vi "Parameter Analyzer Time-IDX_Download.vi"(2 "Error In (no error)":errorcluster, 3 "Trace (variable) name":string, 4 "VISA session":refnum<visa-resource-name>) -> (0 "Error Out":errorcluster, 1 "Trace":dbl[](array[numeric]) format="%^.3e")   [LabVIEW 2014]
uses:
  <instrlib>/Agilent 415X Series/Agilent 415X Series.lvlib
panel:
  # "LICENSED MATERIALS – PROPERTY OF IBM\nCopyright IBM Corp. 2016,\nALL RIGHTS RESERVED"
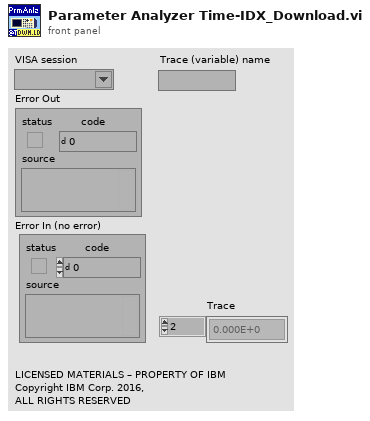
[diagram p1: front panel]
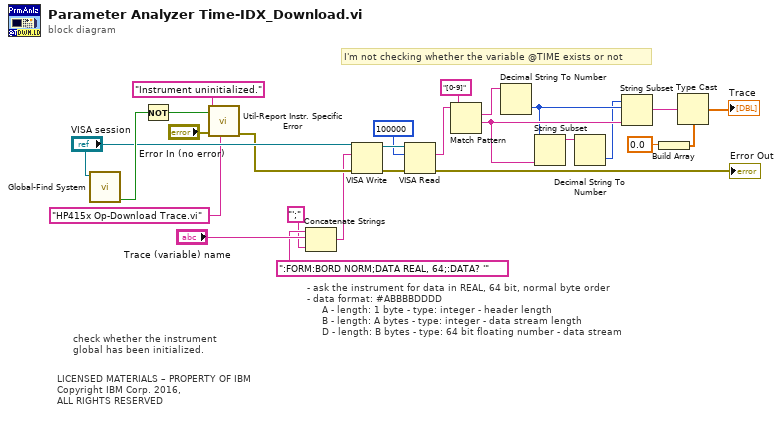
[diagram p0: block diagram]
diagram:
  # "LICENSED MATERIALS – PROPERTY OF IBM\nCopyright IBM Corp. 2016,\nALL RIGHTS RESERVED"
  # "I'm not checking whether the variable @TIME exists or not"
  # "- ask the instrument for data in REAL, 64 bit, normal byte order\n- data format: #ABBBBDDDD \n     A - length: 1 byte - type: integer - header length\n     B - length: A bytes - type: integer - data stream length\n     D - length: B bytes - type: 64 bit floating number - data stream"
  # "check whether the instrument\nglobal has been initialized."
  n1 = call <instrlib>:"Global-Find System.vi"("VISA session"="VISA session") -> ("found"=w25:bool)  [unwired: 10 out]
  n2 = Not(x=w25) -> (.not. x?=w24:bool)
  n3 = call <instrlib>:"Util-Report Instr. Specific Error.vi"("source"="HP415x Op-Download Trace.vi", "error in (no error)"="Error In (no error)", "error message"="Instrument uninitialized.", "new error"=w24) -> ("error out"=w21:errorcluster)  [unwired: 1 in, 6 out]
  n4 = Concatenate Strings(":FORM:BORD NORM;DATA REAL, 64;:DATA? '", "Trace (variable) name", "';") -> (w12:string)
  n5 = VISA Write(VISA resource name="VISA session", write buffer=w12, error in (no error)=w21) -> (VISA resource name out=w16:refnum<visa-resource-name>, error out=w15:errorcluster)  [unwired: 1 out]
  n6 = VISA Read(VISA resource name=w16, byte count=100000, error in (no error)=w15) -> (read buffer=w1:string, error out=→"Error Out":errorcluster)  [unwired: 2 out]
  n7 = Match Pattern(string=w1, regular expression="[0-9]") -> (match substring=w10:string, after substring=w8:string)  [unwired: 3 out]
  n8 = Decimal String To Number(string=w10) -> (number=w7:i32)  [unwired: 3 out]
  n9 = String Subset(string=w8, length (rest)=w7) -> (substring=w6:string)  [unwired: 1 out]
  n10 = Decimal String To Number(string=w6) -> (number=w5:i32)  [unwired: 3 out]
  n11 = String Subset(string=w8, offset (0)=w7, length (rest)=w5) -> (substring=w3:string)
  n12 = Build Array(0.0) -> (w4:dbl[])
  n13 = Type Cast(type=w4, x=w3) -> (*(type *) &x=→"Trace":dbl[])
